vi "File Manager Operations.vi"(7 "Destination (\"\")":string, 8 "error in (no error)":errorcluster, 9 "Source (\"D:\\user\\data\")":string="D:\\user\\data", 10 "Operation (New Folder)":i32(ring) items=["New Folder", "Copy", "Rename", "Delete File", "Delete Directory", "Change Directory", "Change Drive"], 11 "VISA resource name":refnum<visa-resource-name>) -> (0 "error out":errorcluster, 3 "VISA resource name out":refnum<visa-resource-name>)   [LabVIEW 2015, in "Rohde&Schwarz CMXP Base.lvlib"]
doc: "The MMEMory (mass memory) subsystem VI provides commands which allow for access to the storage media of the instrument and for storing and loading various instrument settings.\nThe File to be Printed/Plotted command stores the HCOPy outputs in a file. The various drives can be addressed via the mass storage unit specifier <msus> using the conventional DOS syntax. The internal hard disk is addressed by \"C:\", the floppy-disk drive installed by \"A:\". The file names <file_name> are indicated as string parameters with the commands being enclosed in quotation marks. They correspond to the DOS conventions.\nDOS file names consist of max. 8 ASCII characters and an extension of up to three characters separated from the file name by a colon \".\" Both, the colon and the extension are optional. The colon is not part of the file name. DOS file names do not differ between uppercase and lowercase notation. All letters and digits are permitted as well as the special characters \"_\", \"^\", \"$\", \"~\", \"!\", \"#\", \"%\", \"&\", \"-\", \"{\",\"}\", \"(\", \")\", \"@\" and \"' \". Reserved file names are CLOCK$, CON, AUX, COM1 to COM4, LPT1 to LPT3, NUL and PRN. The two characters \"*\" and \"?\" have the VI of so-called \"wildcards\", i.e., they are variables for selection of several files. The question mark \"?\" replaces exactly one character which may be any, the asterisk means any of the remaining characters in the file name. \"*.*\" thus means all files in a directory.\n\nAttributes:\nRSCMXPBASE_ATTR_CREATE_DIRECTORY\nRSCMXPBASE_ATTR_COPY_FILE\nRSCMXPBASE_ATTR_MOVE\nRSCMXPBASE_ATTR_DELETE_FILE\nRSCMXPBASE_ATTR_DELETE_DIRECTORY\nRSCMXPBASE_ATTR_EDIT_PATH\nRSCMXPBASE_ATTR_CHANGE_DRIVE\n\nRemote-control commands:\nMMEMory:MDIRectory\nMMEMory:COPY\nMMEMory:MOVE\nMMEMory:DELete\nMMEMory:RDIRectory\nMMEMory:CDIRectory\nMMEMory:MSIS"
uses:
  <instrlib>/Rohde&Schwarz CMXP Base/Rohde&Schwarz CMXP Base.lvlib
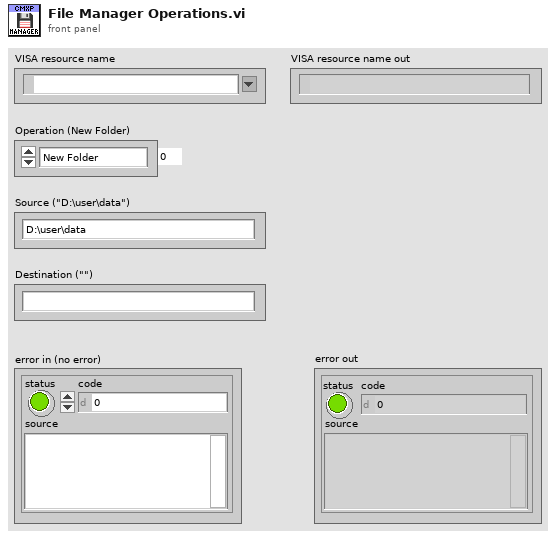
[diagram p1: front panel]
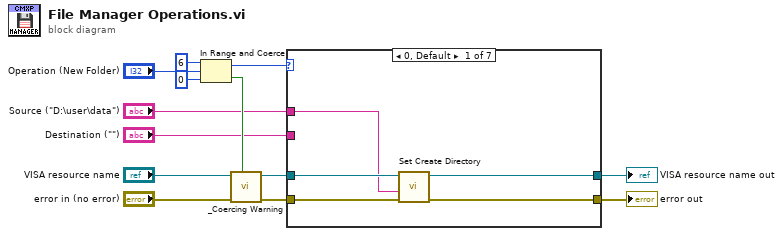
[diagram p0: block diagram]
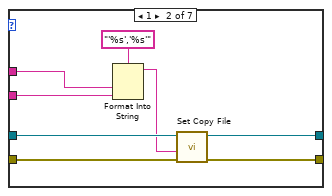
[diagram p2: hidden frame]
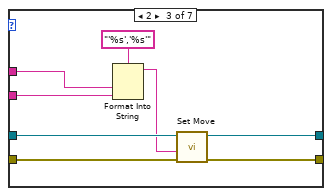
[diagram p3: hidden frame]
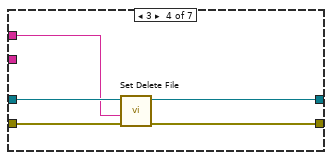
[diagram p4: hidden frame]
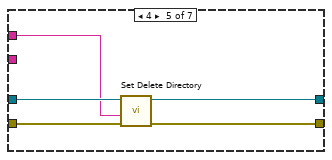
[diagram p5: hidden frame]
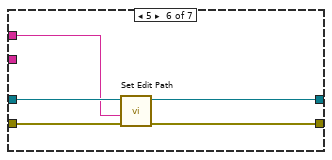
[diagram p6: hidden frame]
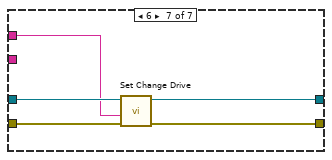
[diagram p7: hidden frame]
diagram:
  n1 = In Range and Coerce(upper limit=6, x="Operation (New Folder)", lower limit=0) -> (coerced(x)=w2:i32, In Range?=w10:bool)
  n2 = call <instrlib>:"_Coercing Warning.vi"("In Range?"=w10, "error in (no error)"="error in (no error)", "VISA resource name"="VISA resource name") -> ("error out"=w6:errorcluster, "VISA resource name out"=w5:refnum<visa-resource-name>)  [unwired: 7 in]
  n3 = case shown="0, Default" w2 {
    tunnel: "Source (\"D:\\user\\data\")" -> [w14 w19 w27 w35 w40 w45 w50]
    tunnel: w6 -> [w18 w26 w34 w39 w44 w49 w54]
    tunnel: w5 -> [w17 w25 w33 w38 w43 w48 w53]
    tunnel: [w16 w24 w32 w37 w42 w47 w52] -> w4
    tunnel: [w15 w23 w31 w36 w41 w46 w51] -> w3
    tunnel: "Destination (\"\")" -> [_ w21 w29 _ _ _ _]
    frame 0, Default {
      n4 = call "Set Create Directory"("error in (no error)"=w18, "Create Directory ()"=w14, "instrument handle"=w17) -> ("error out"=w16:errorcluster, "instrument handle out"=w15:refnum<visa-resource-name>)  [unwired: 7 in]
    }
    frame 1 {
      n5 = Format Into String(format string="'%s','%s'", w19, w21) -> (resulting string=w20:string)  [unwired: 2 in, 1 out]
      n6 = call "Set Copy File"("error in (no error)"=w26, "Copy File ()"=w20, "instrument handle"=w25) -> ("error out"=w24:errorcluster, "instrument handle out"=w23:refnum<visa-resource-name>)  [unwired: 7 in]
    }
    frame 2 {
      n7 = Format Into String(format string="'%s','%s'", w27, w29) -> (resulting string=w28:string)  [unwired: 2 in, 1 out]
      n8 = call "Set Move"("error in (no error)"=w34, "Move ()"=w28, "instrument handle"=w33) -> ("error out"=w32:errorcluster, "instrument handle out"=w31:refnum<visa-resource-name>)  [unwired: 7 in]
    }
    frame 3 {
      n9 = call "Set Delete File"("error in (no error)"=w39, "Delete File ()"=w35, "instrument handle"=w38) -> ("error out"=w37:errorcluster, "instrument handle out"=w36:refnum<visa-resource-name>)  [unwired: 7 in]
    }
    frame 4 {
      n10 = call "Set Delete Directory"("error in (no error)"=w44, "Delete Directory ()"=w40, "instrument handle"=w43) -> ("error out"=w42:errorcluster, "instrument handle out"=w41:refnum<visa-resource-name>)  [unwired: 7 in]
    }
    frame 5 {
      n11 = call "Set Edit Path"("error in (no error)"=w49, "Edit Path ()"=w45, "instrument handle"=w48) -> ("error out"=w47:errorcluster, "instrument handle out"=w46:refnum<visa-resource-name>)  [unwired: 7 in]
    }
    frame 6 {
      n12 = call "Set Change Drive"("error in (no error)"=w54, "Change Drive ()"=w50, "instrument handle"=w53) -> ("error out"=w52:errorcluster, "instrument handle out"=w51:refnum<visa-resource-name>)  [unwired: 7 in]
    }
  }
  "error out" <- w4
  "VISA resource name out" <- w3
